vi "Plot Boxplot Regression.vi"(6 "Config":T1={"title"="", "xlabel"="feaf", "ylabel"="faef", "color"="red", "grid"=TRUE, "xlim"=[], "ylim"=[]}, 7 "Save path":path=path "C:/Users/bogum/OneDrive/Dokumenty/Git/LabVIEW Python Ploter/LabVIEW_python_ploter.py", 8 "error in (no error)":errorcluster, 9 "X positions":dbl[](array[numeric])=[0.0, 1.0, 2.0, 3.0, 4.0], 10 "Data Groups":dbl[][](array[numeric])=[[1.0, 1.0, 1.0, 1.0, nan], [20.0, 2.0, 2.0, 2.0, 2.0], [3.0, 4.0, 5.0, 6.0, 7.0], [1.0, 1.0, 1.0, 1.0, 1.0], [2.0, 2.0, 2.0, 2.0, 2.0]], 11 "PythonPlotter in":refnum<class "PythonPlotter.lvclass">) -> (0 "error out":errorcluster, 3 "PythonPlotter out":refnum<class "PythonPlotter.lvclass">)   [LabVIEW 2024, in "PythonPlotter.lvclass"]
uses:
  PythonPlotter.lvclass
  PythonPlotter.lvclass/PythonPlotter.ctl
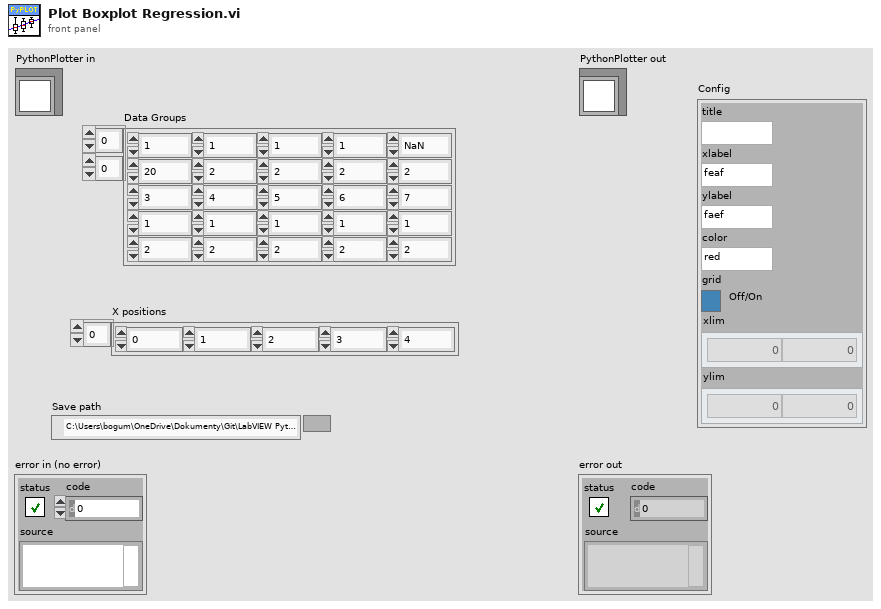
[diagram p1: front panel]
types:
  T1 = cluster{"title":string, "xlabel":string, "ylabel":string, "color":string, "grid":bool, "xlim":dbl[], "ylim":dbl[]}
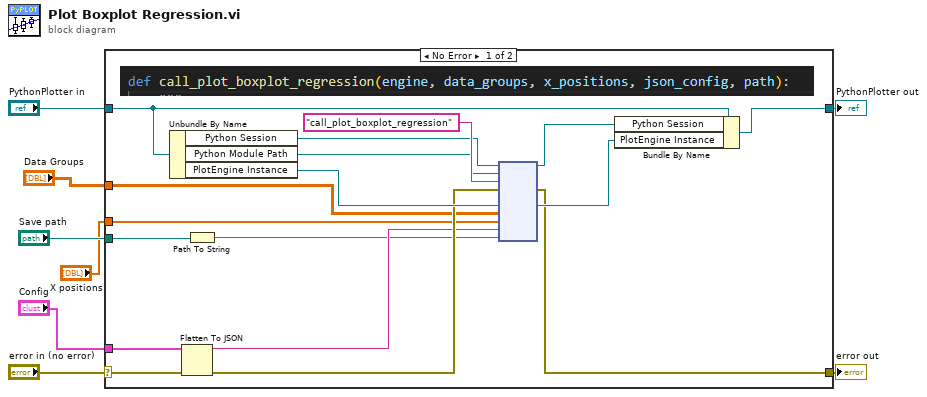
[diagram p0: block diagram]
diagram:
  n1 = case shown="No Error" "error in (no error)" {
    selector: "error in (no error)" -> [w13 w27]
    tunnel: [w14 w27] -> w7
    tunnel: [w15 w26] -> w5
    tunnel: "PythonPlotter in" -> [w16 w26]
    tunnel: "Config" -> [w12 _]
    tunnel: "Save path" -> [w11 _]
    tunnel: "Data Groups" -> [w10 _]
    tunnel: "X positions" -> [w9 _]
    frame No Error {
      n2 = Unbundle By Name(w16) -> ("Python Session"=w24:refnum<k35>, "Python Module Path"=w23:path, "PlotEngine Instance"=w22:refnum<k38>)
      n3 = Flatten To JSON(anything=w12, error in (no error)=w13) -> (JSON string=w20:string, 11:w21:errorcluster)  [unwired: 1 in]
      n4 = Path To String(path=w11) -> (string=w19:string)
      n5 = node(w24, w23, "call_plot_boxplot_regression" ("function name"), w21, w22, w10, w9, w20, w19) -> (w18:refnum<k35>, w14:errorcluster, w17:refnum<k38>)  [unwired: 6 in, 2 out]
      n6 = Bundle By Name(cluster=w16, "Python Session"=w18, "PlotEngine Instance"=w17) -> (w15:refnum<class "PythonPlotter.lvclass">)
    }
    frame Error {
    }
  }
  "error out" <- w7
  "PythonPlotter out" <- w5
